vi "ScriptManager.vi"() -> ()   [LabVIEW 2021]
uses:
  <vilib>/Utility/miscctls.llb/LVSelectionTypeDef.ctl
  <vilib>/event_ctls.llb/eventvkey.ctl
  <vilib>/Utility/miscctls.llb/LVRectTypeDef.ctl
  <vilib>/Platform/browser.llb/Open URL in Default Browser (string).vi
  <vilib>/regexp/Match Regular Expression.xnode
  ScriptManager/ScriptManager.lvlib
  lib/UI/TreeControl/TreeControlLib.lvlib
panel:
  out "Dirty":refnum<vi>
  out "InifilePath":path
  out "PreviousSaveMode":string
  out "Allowed Parent Child":set{cluster{"Parent":i32, "Child":i32}}(c389)
  out "VKey":T1
  out "Edit Mode":enum16{"unknown", "inserting", "deleting"}(ring)
  out "Text.Selection":T2
  out "RedoBuffer":string[](array[string])
  out "UndoBuffer":string[](array[string])
  out "ItemTagToName":map{string, string}(c390)
  out "editor refs":refnum<vi>[](array[refnum])
  in  "Show Editor":bool
  in  "Tree":string(tree) caption="Tree (use right click menu to edit)"
  out "Last Modified":refnum<vi>
  in  "Exec":bool
  out "Modified":string
  in  "Description":string
  in  "Title":string
  in  "VI Property Picker":bool
  in  "Script":string
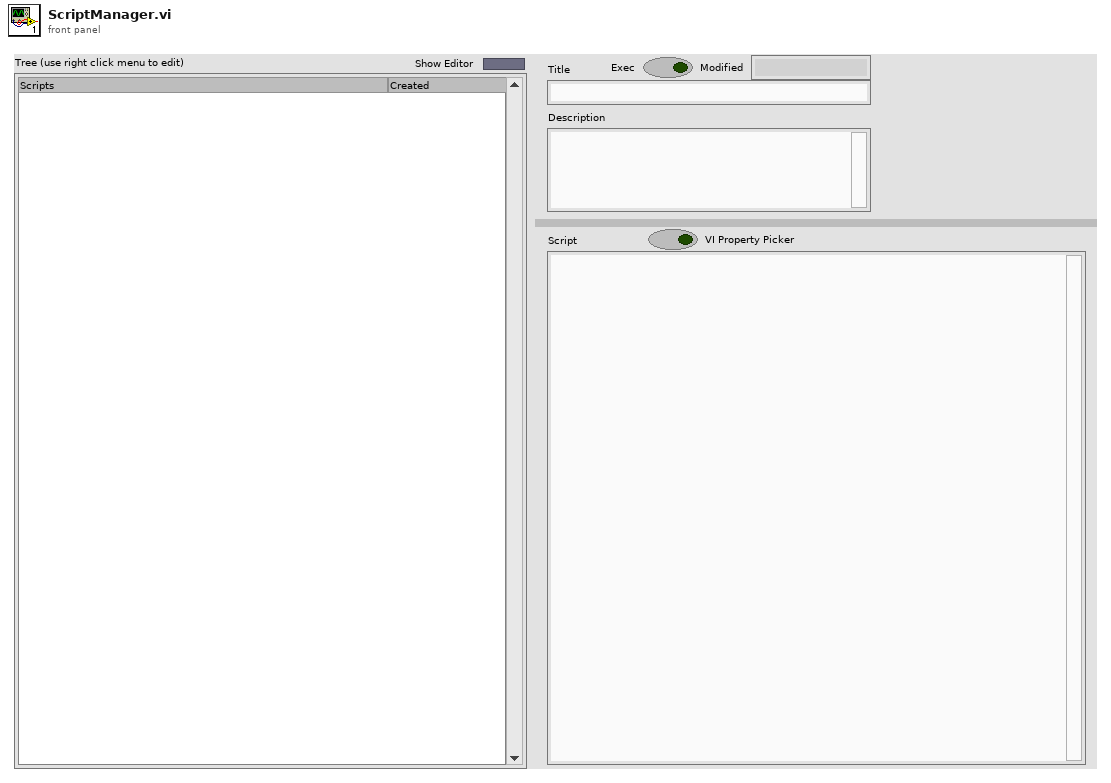
[diagram p1: front panel]
types:
  T1 = typedef "eventvkey.ctl" = enum16{"ASCII", "Enter", "Return", "Shift", "Ctrl", "Alt", "Cmd", "Opt", "Caps", "NumLock", "Clear", "Break", "Up", "Down", "Left", "Right", "Insert", "Delete", "Home", "End", "PageUp", "PageDown", "Escape", "Help", "Pause", "ScrollLock", "F1", "F2", "F3", "F4", "F5", "F6", "F7", "F8", "F9", "F10", "F11", "F12", "F13", "F14", "F15", "F16", "F17", "F18", "F19", "F20", "F21", "F22", "F23", "F24", "Play", "VolumeUp", "VolumeDown", "Mute", "Two Byte Char"}
  T2 = typedef "LVSelectionTypeDef.ctl" = cluster{"Selection Start":u32, "Selection End":u32}
  T3 = cluster{"Name":string, "Include Shift Key?":bool, "Include Ctrl Key?":bool, "Shortcut Key":string}[]
  T4 = enum32{"Invalid", "Standard", "Closed", "Hidden", "Minimized", "Maximized"}
  T5 = enum16{"open", "replace", "create", "open or create", "replace or create", "replace or create with confirmation"}
  T6 = typedef "LVRectTypeDef.ctl" = cluster{"Left":i16, "Top":i16, "Right":i16, "Bottom":i16}
  T7 = enum8{"Enabled", "Disabled", "Disabled and Grayed Out"}
  T8 = cluster{"[0]":i32, "[1]":i32, "[2]":i32, "[3]":i32, "[4]":i32}
  T9 = enum16{"Sticks Top/Left", "Sticks Bottom/Right", "Proportional"}
  T10 = typedef "LVPoint32TypeDef.ctl" = cluster{"Horizontal":i32, "Vertical":i32}
  T11 = typedef "LVRowAndColumnTypeDef.ctl" = cluster{"Row":i32, "Column":i32}
  T12 = typedef "lveventtype.ctl" = enum32{"Null", "Timeout", "Annotation Menu Selection", "Annotation Menu Selection?", "App Instance Close", "App Instance Close?", "Autoscale Range Change", "Bookmark Info Change", "Cell Edit", "Cell Edit?", "Cursor Grab", "Cursor Grab?", "Cursor Menu Selection", "Cursor Menu Selection?", "Cursor Move", "Cursor Release", "Data Change", "Direction Change", "Display State Change", "Drag Ended", "Drag Enter", "Drag Leave", "Drag Over", "Drag Source Update", "Drag Starting", "Drag Starting?", "Drop", "Exec State Change", "Key Down", "Key Down?", "Key Repeat", "Key Repeat?", "Key Up", "Listbox Double Click", "Menu Activation?", "Menu Selection (App)", "Menu Selection? (App)", "Menu Selection (User)", "Mouse Down", "Mouse Down?", "Mouse Enter", "Mouse Leave", "Mouse Move", "Mouse Up", "Mouse Wheel", "NI Security User Change (App)", "Pane Size", "Panel Close", "Panel Close?", "Panel Resize", "Plot Attribute Change", "Scale Range Change", "Shortcut Menu Activation?", "Shortcut Menu Selection (App)", "Shortcut Menu Selection? (App)", "Shortcut Menu Selection (User)", "Tree Double Click", "Tree Drag", "Tree Drag?", "Tree Drop", "Tree Drop?", "Tree Item Close", "Tree Item Close?", "Tree Item Open", "Tree Item Open?", "User Event", "Value Change"}
  T13 = cluster{"Shift":bool, "Ctrl":bool, "Alt":bool, "Cmd":bool, "Opt":bool}
  T14 = cluster{"Tag":string, "Symbol Index":i32, "Indent Level":i32, "Disabled?":bool, "In Symbol?":bool, "Position":enum16{"Top", "Center", "Bottom"}}
  T15 = enum32{"Bad", "Idle", "Run top level", "Running"}
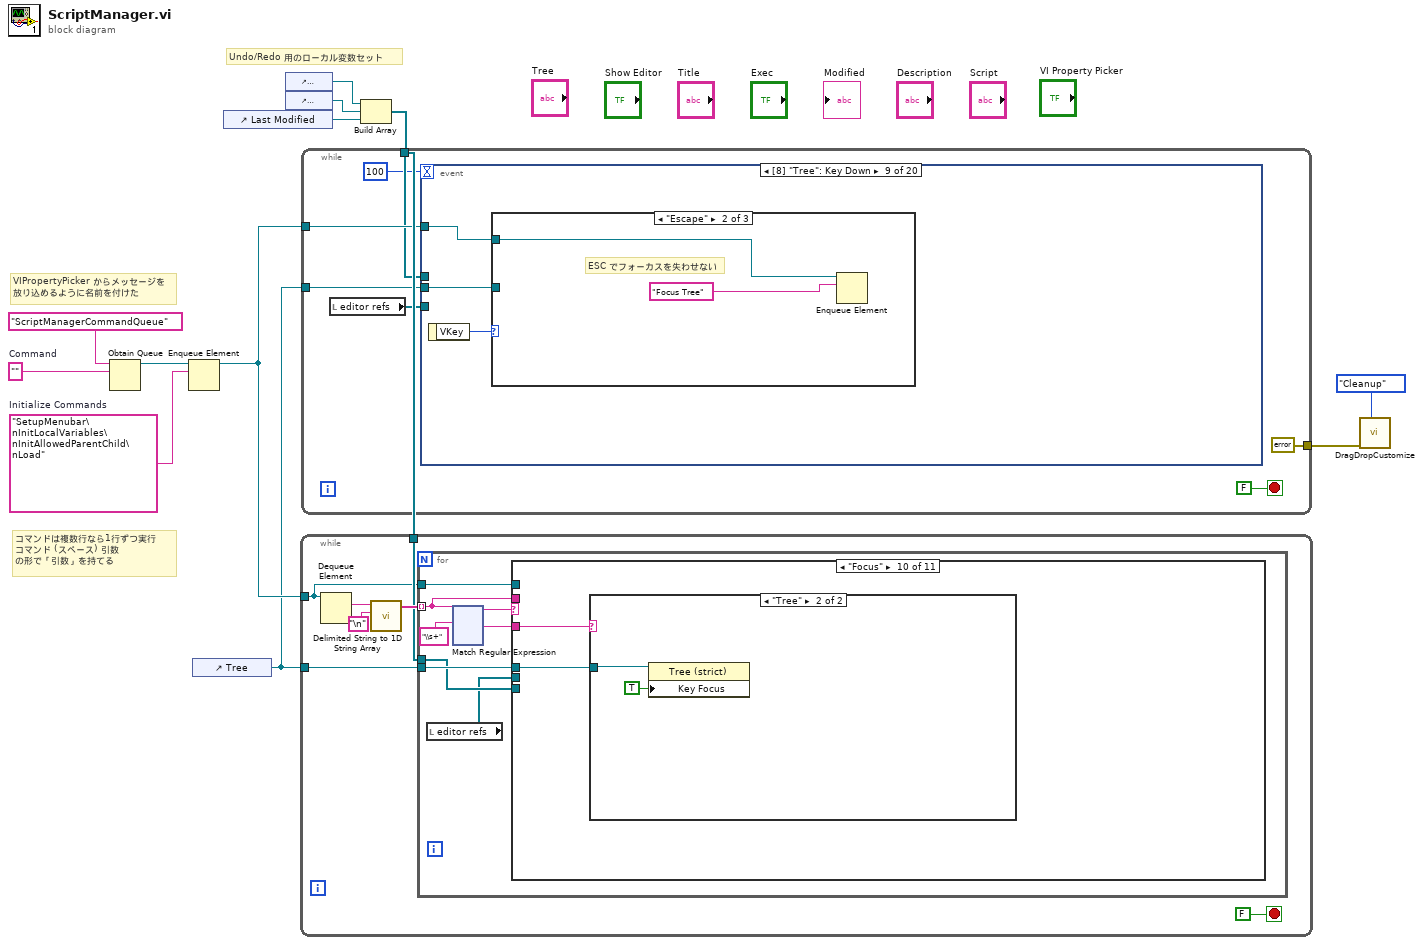
[diagram p0: block diagram]
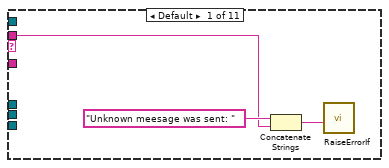
[diagram p2: hidden frame]
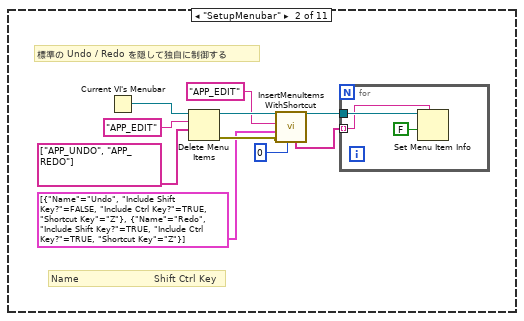
[diagram p3: hidden frame]
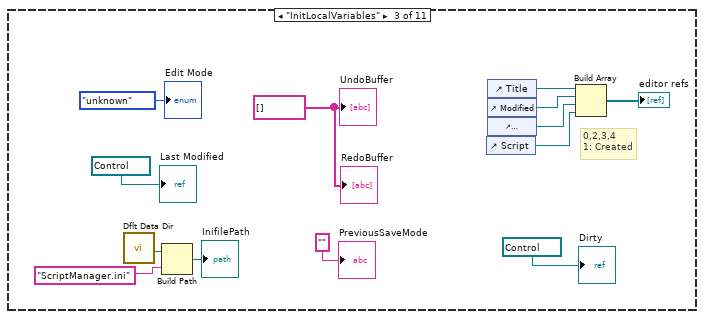
[diagram p4: hidden frame]
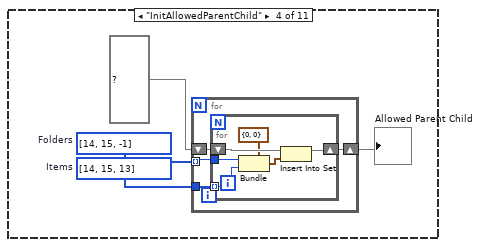
[diagram p5: hidden frame]
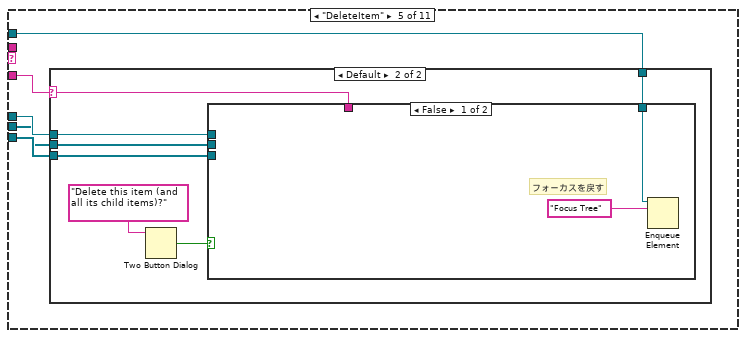
[diagram p6: hidden frame]
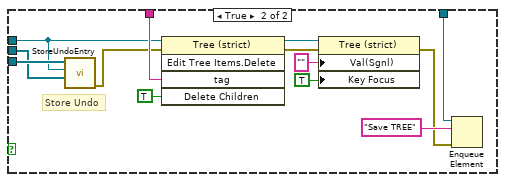
[diagram p8: hidden frame]
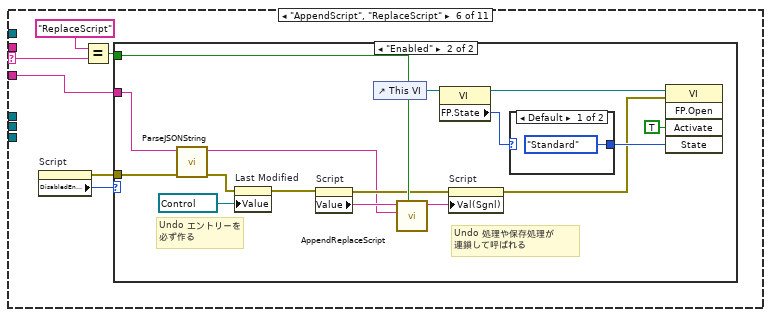
[diagram p9: hidden frame]
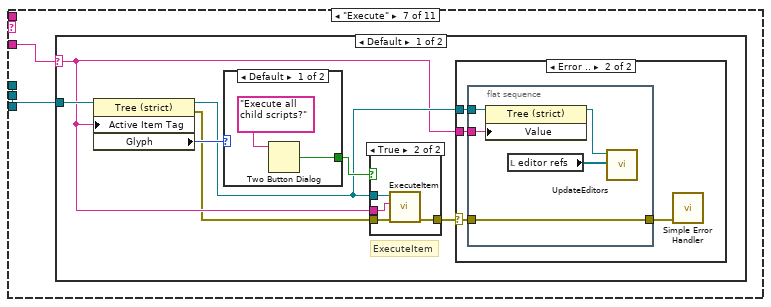
[diagram p12: hidden frame]
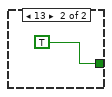
[diagram p15: hidden frame]
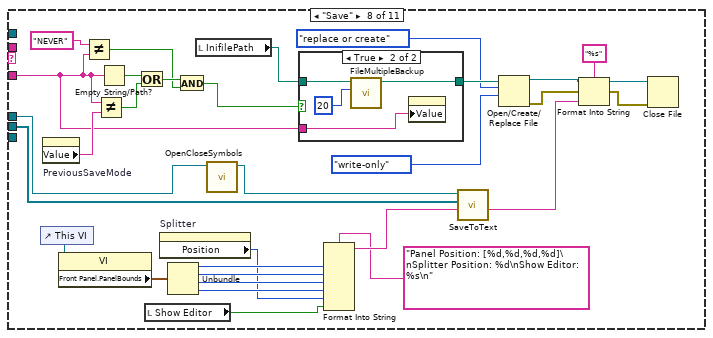
[diagram p17: hidden frame]
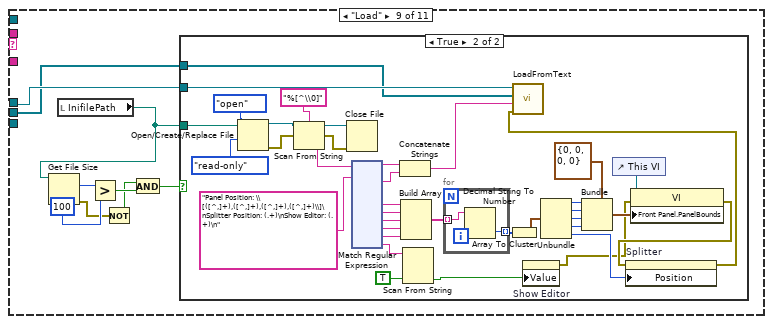
[diagram p19: hidden frame]
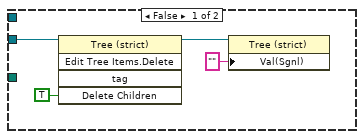
[diagram p20: hidden frame]
diagram:
  w7 = "SetupMenubar\nInitLocalVariables\nInitAllowedParentChild\nLoad"  # Initialize Commands
  w10 = ""  # Command
  # "Undo/Redo 用のローカル変数セット"
  # "コマンドは複数行なら1行ずつ実行\nコマンド (スペース) 引数\nの形で「引数」を持てる"
  # "VIPropertyPicker からメッセージを\n放り込めるように名前を付けた"
  n1 = Obtain Queue(name (unnamed)="ScriptManagerCommandQueue", element data type=w10) -> (queue out=w9:refnum<queue>)  [unwired: 3 in, 2 out]
  n2 = Enqueue Element(queue=w9, element=w7) -> (queue out=w8:refnum<queue>)  [unwired: 2 in, 2 out]
  n3 = control-ref of="Tree"() -> (w1:refnum<vi>)
  n4 = control-ref of="Last Modified"() -> (w2:refnum<vi>)
  n5 = control-ref of="UndoBuffer"() -> (w4:refnum<vi>)
  n6 = control-ref of="RedoBuffer"() -> (w5:refnum<vi>)
  n7 = Build Array(w4, w5, w2) -> (w3:refnum<vi>[])
  n8 = while {
    tunnel: w8 -> [w13]
    tunnel: w1 -> [w16]
    tunnel: w3 -> [w14]
    stop <- FALSE stop-if-true
    n9 = Dequeue Element(queue=w13) -> (element=w18:string)  [unwired: 2 in, 3 out]
    n10 = call <vilib>:"Delimited String to 1D String Array.vi"("delimiter"="\n", "delimited string"=w18) -> ("string array"=w17:string[])  [unwired: 9 in]
    n11 = for {
      tunnel: w17 -> [w20] mode=indexing
      tunnel: w16 -> [w24]
      tunnel: w14 -> [w23]
      tunnel: w13 -> [w22]
      n12 = local read "editor refs"() -> (w21:refnum<vi>[])
      n13 = xnode "Match Regular Expression"("input string"=w20, "regular expression"="\\s+") -> ("before match"=w26:string, "after match"=w25:string)  [unwired: 4 in, 3 out]
      n14 = case shown="\"Focus\"" w26 {
        selector: w26 -> [_ _ _ _ _ w217 _ _ _ _ _]
        tunnel: w25 -> [_ _ _ _ w192 w219 w240 w265 _ w478 _]
        tunnel: w24 -> [_ _ _ _ w191 _ w239 w269 w306 w477 _]
        tunnel: w20 -> [w146 _ _ _ _ _ _ _ _ _ _]
        tunnel: w23 -> [_ _ _ _ w190 _ _ _ _ _ _]
        tunnel: w21 -> [_ _ _ _ w189 _ _ w288 w305 _ _]
        tunnel: w22 -> [_ _ _ _ w188 _ _ _ _ _ _]
        frame Default {
          n15 = Concatenate Strings("Unknown meesage was sent: ", w146) -> (w145:string)
          n16 = call "RaiseErrorIf.vi"("error message"=w145) -> ()  [unwired: 10 in, 1 out]
        }
        frame "SetupMenubar" {
          # "標準の Undo / Redo を隠して独自に制御する"
          # "Name                         Shift Ctrl Key"
          n17 = Current VI's Menubar() -> (w153:refnum<k9>)
          n18 = Delete Menu Items(7:string[] ["APP_UNDO", "APP_REDO"], 8:"APP_EDIT", 9:w153) -> (0:w154:errorcluster, 3:w155:refnum<k9>)  [unwired: 1 in]
          n19 = call "InsertMenuItemsWithShortcut.vi"("Insert After (last)"=0, "error in (no error)"=w154, "Sub Items"=T3 [{"Name"="Undo", "Include Shift Key?"=FALSE, "Include Ctrl Key?"=TRUE, "Shortcut Key"="Z"}, {"Name"="Redo", "Include Shift Key?"=TRUE, "Include Ctrl Key?"=TRUE, "Shortcut Key"="Z"}] ("Menu Short Cut"), "Target Tag"="APP_EDIT", "menu ref"=w155) -> ("menu ref out"=w156:refnum<k9>, "Sub Item Names"=w157:string[])  [unwired: 3 in, 2 out]
          n20 = for {
            tunnel: w156 -> [w160]
            tunnel: w157 -> [w159] mode=indexing
            n21 = Set Menu Item Info(7:w159, 9:FALSE ("enabled"), 11:w160) -> ()  [unwired: 4 in, 2 out]
          }
        }
        frame "InitLocalVariables" {
          w166 = string[] [] ("UndoBuffer")
          # "0,2,3,4\n1: Created"
          n22 = call <vilib>:"Dflt Data Dir.vi"() -> ("App:Default Data Directory"=w164:path)
          n23 = Build Path(base path=w164, name or relative path="ScriptManager.ini") -> (appended path=→"InifilePath":path)
          n24 = control-ref of="Script"() -> (w169:refnum<vi>)
          n25 = control-ref of="Title"() -> (w168:refnum<vi>)
          n26 = control-ref of="Modified"() -> (w167:refnum<vi>)
          n27 = control-ref of="Description"() -> (w170:refnum<vi>)
          n28 = Build Array(w168, w167, w170, w169) -> (→"editor refs":refnum<vi>[])
          "Edit Mode" <- enum16{"unknown", "inserting", "deleting"}."unknown"
          "Last Modified" <- refnum<vi> refnum ("Last Modified")
          "UndoBuffer" <- w166
          "RedoBuffer" <- w166
          "PreviousSaveMode" <- "" ("PreviousSaveMode")
          "Dirty" <- refnum<vi> refnum ("Dirty")
        }
        frame "InitAllowedParentChild" {
          w177 = i32[] [14, 15, -1]  # Folders
          w176 = i32[] [14, 15, 13]  # Items
          n29 = for {
            tunnel: w177 -> [w179] mode=indexing
            tunnel: w176 -> [w181]
            shift-right: [w178] -> w174
            shift-left: set{cluster{"Parent":i32, "Child":i32}} {} ("Allowed Parent Child") -> [w180]
            n30 = for {
              tunnel: w181 -> [w187] mode=indexing
              tunnel: w179 -> [w186]
              shift-right: [w182] -> w178
              shift-left: w180 -> [w184]
              n31 = Bundle(cluster=cluster{"Parent":i32, "Child":i32} {"Parent"=0, "Child"=0} ("element"), "Parent"=w186, "Child"=w187) -> (w185:cluster{"Parent":i32, "Child":i32})
              n32 = Insert Into Set(10:w185, 11:w184) -> (3:w182:set{cluster{"Parent":i32, "Child":i32}})  [unwired: 1 out]
            }
          }
          "Allowed Parent Child" <- w174
        }
        frame "DeleteItem" {
          n33 = case shown="Default" w192 {
            selector: w192 -> [_ w198]
            tunnel: w191 -> [_ w199]
            tunnel: w190 -> [_ w195]
            tunnel: w189 -> [_ w194]
            tunnel: w188 -> [_ w193]
            frame "" {
            }
            frame Default {
              n34 = Two Button Dialog(message="Delete this item (and all its child items)?") -> (T button?=w196:bool)  [unwired: 2 in]
              n35 = case shown="False" w196 {
                tunnel: w199 -> [_ w207]
                tunnel: w198 -> [_ w213]
                tunnel: w195 -> [_ w208]
                tunnel: w194 -> [_ w206]
                tunnel: w193 -> [w200 w202]
                frame False {
                  # "フォーカスを戻す"
                  n36 = Enqueue Element(queue=w200, element="Focus Tree") -> ()  [unwired: 2 in, 3 out]
                }
                frame True {
                  # "Store Undo"
                  n37 = call "StoreUndoEntry.vi"("editor refs"=w206, "Tree"=w207, "UndoBuffer"=w208) -> ("error out"=w209:errorcluster)  [unwired: 8 in]
                  n38 = invoke class="Tree (strict)" method="Edit Tree Items.Delete"(reference=w207, error in=w209, "tag"=w213, "Delete Children"=TRUE ("Delete Children?")) -> (reference out=w212:refnum<vi>, error out=w211:errorcluster)  [unwired: 1 in, 3 out]
                  n39 = property class="Tree (strict)"(reference=w212, error in=w211, "Val(Sgnl)"="" ("Value"), "Key Focus"=TRUE) -> (error out=w203:errorcluster)  [unwired: 1 out]
                  n40 = Enqueue Element(queue=w202, element="Save TREE", error in (no error)=w203) -> ()  [unwired: 1 in, 3 out]
                }
              }
            }
          }
        }
        frame "AppendScript", "ReplaceScript" {
          n41 = property on="Script" class="Str"() -> (error out=w218:errorcluster, "DisabledEnum"=w220:T7)  [unwired: 2 in, 1 out]
          n42 = Equal?(x="ReplaceScript", y=w217) -> (x = y?=w215:bool)
          n43 = case shown="\"Enabled\"" w220 {
            tunnel: w219 -> [_ w236]
            tunnel: w218 -> [_ w234]
            tunnel: w215 -> [_ w227]
            frame Default {
            }
            frame "Enabled" {
              # "Undo エントリーを\n必ず作る"
              # "Undo 処理や保存処理が\n連鎖して呼ばれる"
              n44 = call "ParseJSONString.vi"("error in (no error)"=w234, "JSON string"=w236) -> ("error out"=w225:errorcluster, "string"=w221:string)  [unwired: 8 in]
              n45 = property on="Last Modified" class="LVObjRef (strict)"(error in=w225, "Value"=refnum<vi> refnum ("Last Modified")) -> (error out=w222:errorcluster)  [unwired: 1 in, 1 out]
              n46 = property on="Script" class="Str"(error in=w222) -> (error out=w226:errorcluster, "Value"=w228:string)  [unwired: 1 in, 1 out]
              n47 = control-ref of="This VI"() -> (w233:refnum<vi>)
              n48 = call "AppendReplaceScript.vi"("Replace"=w227, "New Script"=w221, "Old Script"=w228) -> ("Result"=w235:string)  [unwired: 8 in]
              n49 = property class="VI"(reference=w233) -> (reference out=w231:refnum<vi>, "FP.State"=w230:T4)  [unwired: 1 in, 1 out]
              n50 = property on="Script" class="Str"(error in=w226, "Val(Sgnl)"=w235) -> (error out=w223:errorcluster)  [unwired: 1 in, 1 out]
              n51 = case shown="Default" w230 {
                selector: w230 -> [_ w238]
                tunnel: [T4."Standard" ("State") w238] -> w229
                frame Default {
                }
                frame "Standard", "Maximized" {
                }
              }
              n52 = invoke class="VI" method="FP.Open"(reference=w231, error in=w223, "Activate"=TRUE ("Activate?"), "State"=w229) -> ()  [unwired: 1 in, 5 out]
            }
          }
        }
        frame "Execute" {
          n53 = case shown="Default" w240 {
            selector: w240 -> [w242 _]
            tunnel: w239 -> [w247 _]
            frame Default {
              # "ExecuteItem"
              n54 = property class="Tree (strict)"(reference=w247, "Active Item Tag"=w242) -> (reference out=w243:refnum<vi>, error out=w241:errorcluster, "Glyph"=w246:i32)  [unwired: 1 in]
              n55 = case shown="Default" w246 {
                tunnel: [w262 TRUE ("T button?")] -> w245
                frame Default {
                  n56 = Two Button Dialog(message="Execute all child scripts?") -> (T button?=w262:bool)  [unwired: 2 in]
                }
                frame 13 {
                }
              }
              n57 = case shown="True" w245 {
                tunnel: w243 -> [_ w261]
                tunnel: w242 -> [_ w260]
                tunnel: [w257 w259] -> w244
                tunnel: w241 -> [w257 w258]
                frame False {
                }
                frame True {
                  n58 = call "ExecuteItem.vi"("error in (no error)"=w258, "Tag"=w260, "TreeControl in"=w261) -> ("error out"=w259:errorcluster)  [unwired: 8 in]
                }
              }
              n59 = case shown="Error .." w244 {
                selector: w244 -> [_ w249]
                tunnel: w243 -> [_ w251]
                tunnel: w242 -> [_ w250]
                frame No Error {
                }
                frame Error {
                  n60 = flat-sequence {
                    tunnel: w251 -> [w256]
                    tunnel: w250 -> [w255]
                    tunnel: w249 -> [w252]
                    tunnel: [w252] -> w248
                    frame #0 {
                      n61 = property class="Tree (strict)"(reference=w256, "Value"=w255) -> (reference out=w254:refnum<vi>)  [unwired: 1 in, 1 out]
                      n62 = local read "editor refs"() -> (w253:refnum<vi>[])
                      n63 = call "UpdateEditors.vi"("Array"=w253, "TreeControl in"=w254) -> ()  [unwired: 9 in, 1 out]
                    }
                  }
                  n64 = call <vilib>:"Simple Error Handler.vi"("error in (no error)"=w248) -> ()  [unwired: 4 in, 5 out]
                }
              }
            }
            frame "" {
            }
          }
        }
        frame "Save" {
          n65 = control-ref of="This VI"() -> (w283:refnum<vi>)
          n66 = property on="PreviousSaveMode" class="Str"() -> ("Value"=w267:string)  [unwired: 2 in, 2 out]
          n67 = property class="VI"(reference=w283) -> ("Front Panel.PanelBounds"=w282:T6)  [unwired: 1 in, 2 out]
          n68 = Not Equal?(x="NEVER", y=w265) -> (x != y?=w270:bool)
          n69 = Not Equal?(x=w265, y=w267) -> (x != y?=w294:bool)
          n70 = Empty String/Path?(string/path=w265) -> (empty?=w295:bool)
          n71 = Or(x=w295, y=w294) -> (x .or. y?=w292:bool)
          n72 = local read "Show Editor"() -> (w276:bool)
          n73 = property on="Splitter" class="Splitter"() -> ("Position"=w277:i32)  [unwired: 2 in, 2 out]
          n74 = Unbundle(w282) -> ("Left"=w281:i16, "Top"=w280:i16, "Right"=w279:i16, "Bottom"=w278:i16)
          n75 = And(x=w292, y=w270) -> (x .and. y?=w271:bool)
          n76 = local read "InifilePath"() -> (w293:path)
          n77 = call "OpenCloseSymbols.vi"("Tree ref"=w269) -> ("Tree ref out"=w268:refnum<vi>)  [unwired: 9 in, 1 out]
          n78 = case shown="True" w271 {
            tunnel: w293 -> [w296 w299]
            tunnel: [w296 w298] -> w291
            tunnel: w265 -> [_ w297]
            frame False {
            }
            frame True {
              n79 = call "FileMultipleBackup.vi"("Number of Backups"=20, "File path"=w299) -> ("File path out"=w298:path)  [unwired: 9 in]
              n80 = property on="PreviousSaveMode" class="Str"("Value"=w297) -> ()  [unwired: 2 in, 2 out]
            }
          }
          n81 = Format Into String(format string="Panel Position: [%d,%d,%d,%d]\nSplitter Position: %d\nShow Editor: %s\n", w281, w280, w279, w278, w277, w276) -> (resulting string=w275:string)  [unwired: 2 in, 1 out]
          n82 = call "SaveToText.vi"("Additional Header"=w275, "editor refs"=w288, "Tree ref"=w268) -> ("String"=w285:string)  [unwired: 7 in, 1 out]
          n83 = Open/Create/Replace File(file path (use dialog)=w291, operation (0:open)=T5."replace or create", access (0:read/write)=enum16{"read/write", "read-only", "write-only"}."write-only") -> (refnum out=w287:refnum<file>, error out=w286:errorcluster)  [unwired: 3 in, 1 out]
          n84 = Format Into String(format string="%s", initial string=w287, error in=w286, w285) -> (resulting string=w273:refnum<file>, error out=w274:errorcluster)
          n85 = Close File(refnum=w273, error in=w274) -> ()  [unwired: 2 out]
        }
        frame "Load" {
          n86 = local read "InifilePath"() -> (w301:path)
          n87 = Get File Size(file=w301) -> (size (in bytes)=w309:i64, 0:w303:errorcluster)  [unwired: 1 in, 1 out]
          n88 = Greater?(x=w309, y=i64 100) -> (0:w307:bool)
          n89 = Not(x=w303) -> (.not. x?=w302:bool)
          n90 = And(x=w302, y=w307) -> (x .and. y?=w304:bool)
          n91 = case shown="True" w304 {
            tunnel: w301 -> [_ w344]
            tunnel: w306 -> [w313 w317]
            tunnel: w305 -> [_ w316]
            frame False {
              n92 = invoke class="Tree (strict)" method="Edit Tree Items.Delete"(reference=w313, "Delete Children"=TRUE ("Delete Children?")) -> (reference out=w312:refnum<vi>)  [unwired: 3 in, 4 out]
              n93 = property class="Tree (strict)"(reference=w312, "Val(Sgnl)"="" ("Value (Signaling)")) -> ()  [unwired: 1 in, 2 out]
            }
            frame True {
              n94 = Open/Create/Replace File(file path (use dialog)=w344, operation (0:open)=T5."open", access (0:read/write)=enum16{"read/write", "read-only", "write-only"}."read-only") -> (refnum out=w347:refnum<file>, error out=w348:errorcluster)  [unwired: 3 in, 1 out]
              n95 = Scan From String("%[^\\0]" ("format string"), w347, w348) -> (w350:refnum<file>, w349:errorcluster, output 1=w341:string)  [unwired: 1 in]
              n96 = Close File(refnum=w350, error in=w349) -> ()  [unwired: 2 out]
              n97 = xnode "Match Regular Expression"("input string"=w341, "regular expression"="Panel Position: \\[([^,]+),([^,]+),([^,]+),([^,]+)\\]\nSplitter Position: (.+)\nShow Editor: (.+)\n" ("format string")) -> ("before match"=w334:string, "after match"=w333:string, "submatch 1"=w340:string, "submatch 2"=w339:string, "submatch 3"=w338:string, "submatch 4"=w337:string, "submatch 5"=w336:string, "submatch 6"=w323:string)  [unwired: 4 in, 3 out]
              n98 = Concatenate Strings(w334, w333) -> (w318:string)
              n99 = Build Array(w340, w339, w338, w337, w336) -> (w335:string[])
              n100 = Scan From String(input string=w323, default 1=TRUE) -> (output 1=w321:bool)  [unwired: 3 in, 3 out]
              n101 = for {
                tunnel: w335 -> [w352] mode=indexing
                tunnel: [w351] -> w332 mode=indexing
                n102 = Decimal String To Number(string=w352) -> (number=w351:i32)  [unwired: 2 in, 1 out]
              }
              n103 = Array To Cluster(array=w332) -> (cluster=w331:T8)
              n104 = property on="Show Editor" class="Bool (strict)"("Value"=w321) -> (error out=w315:errorcluster)  [unwired: 2 in, 1 out]
              n105 = Unbundle(w331) -> ("[0]"=w329:i32, "[1]"=w328:i32, "[2]"=w327:i32, "[3]"=w326:i32, "[4]"=w320:i32)
              n106 = Bundle(cluster=T6 {"Left"=0, "Top"=0, "Right"=0, "Bottom"=0} ("Front Panel Window:Panel Bounds"), "Left"=w329, "Top"=w328, "Right"=w327, "Bottom"=w326) -> (w325:T6)
              n107 = control-ref of="This VI"() -> (w324:refnum<vi>)
              n108 = property class="VI"(reference=w324, error in=w315, "Front Panel.PanelBounds"=w325) -> (error out=w319:errorcluster)  [unwired: 1 out]
              n109 = property on="Splitter" class="Splitter"(error in=w319, "Position"=w320) -> (error out=w314:errorcluster)  [unwired: 1 in, 1 out]
              n110 = call "LoadFromText.vi"("error in"=w314, "String"=w318, "editor refs"=w316, "Tree ref"=w317) -> ()  [unwired: 6 in, 2 out]
            }
          }
        }
        frame "Focus" {
          n111 = case shown="\"Tree\"" w478 {
            tunnel: w477 -> [_ w480]
            frame Default {
            }
            frame "Tree" {
              n112 = property class="Tree (strict)"(reference=w480, "Key Focus"=TRUE) -> ()  [unwired: 1 in, 2 out]
            }
          }
        }
        frame "" {
        }
      }
    }
  }
  n113 = while {
    tunnel: [errorcluster {"status"=FALSE, "code"=0, "source"=""} ("error in (no error)")] -> w11
    tunnel: w8 -> [w485]
    tunnel: w3 -> [w483]
    tunnel: w1 -> [w482]
    stop <- FALSE stop-if-true
    n114 = local read "editor refs"() -> (w484:refnum<vi>[])
    n115 = event shown="[8] \"Tree\": Key Down" {
      selector: _ -> [_ _ _ _ _ _ _ _ _ _ _ _ _ _ _ _ _ _ _ _]
      dyn-events: _ -> [_ _ _ _ _ _ _ _ _ _ _ _ _ _ _ _ _ _ _ _]
      timeout: 100 -> [_ _ _ _ _ _ _ _ _ _ _ _ _ _ _ _ _ _ _ _]
      tunnel: w482 -> [w492 _ _ _ w564 w583 _ w638 w657 w683 _ _ _ w732 _ _ _ _ _ _]
      tunnel: w485 -> [w490 w527 w540 w542 _ w582 _ w636 w658 w679 _ w709 _ w729 _ _ _ w770 w778 _]
      tunnel: w484 -> [w491 _ _ _ _ w578 _ w637 _ w682 _ _ _ w727 _ _ _ _ _ _]
      tunnel: w483 -> [w493 _ _ _ _ w577 _ w639 _ w684 _ _ _ w728 _ _ _ _ _ _]
      event Timeout {
        n116 = event-data() -> ()  [unwired: 1 in, 1 out]
        n117 = local read "Dirty"() -> (w488:refnum<vi>)
        n118 = Not A Number/Path/Refnum?(number/path/refnum=w488) -> (NaN/Path/Refnum?=w489:bool)
        n119 = case shown="False" w489 {
          tunnel: w493 -> [w501 _]
          tunnel: w492 -> [w500 _]
          tunnel: w491 -> [w499 _]
          tunnel: w490 -> [w496 _]
          tunnel: w488 -> [w495 _]
          frame False {
            n120 = local read "Text.Selection"() -> (w497:T2)
            n121 = call "StoreUndoEntry.vi"("Text.Selection"=w497, "Changed Editor"=w495, "editor refs"=w499, "Tree"=w500, "UndoBuffer"=w501) -> ("error out"=w498:errorcluster)  [unwired: 6 in]
            n122 = property class="Tree (strict)"(reference=w500, error in=w498) -> (reference out=w503:refnum<vi>, error out=w502:errorcluster, "Value"=w504:string)
            n123 = local write "Dirty"(refnum<vi> refnum ("Dirty")) -> ()
            n124 = case shown="Default" w504 {
              selector: w504 -> [_ w510]
              tunnel: w503 -> [_ w509]
              tunnel: w502 -> [_ w508]
              tunnel: w496 -> [_ w505]
              frame "" {
              }
              frame Default {
                n125 = Format Date/Time String(time format string (%c)="%Y-%m-%d %H:%M:%S") -> (date/time string=w511:string)  [unwired: 2 in]
                n126 = local read "Description"() -> (w515:string)
                n127 = local read "Script"() -> (w514:string)
                n128 = local read "Title"() -> (w516:string)
                n129 = local write "Modified"(w511) -> ()
                n130 = Build Array(w516, w511, w515, w514) -> (w513:string[])
                n131 = for {
                  shift-right: [w522] -> _
                  shift-left: w509 -> [w524]
                  shift-right: [w523] -> w506
                  shift-left: w508 -> [w521]
                  tunnel: i32[] [0, 2, 3, 4] -> [w520] mode=indexing
                  tunnel: w513 -> [w519] mode=indexing
                  tunnel: w510 -> [w518]
                  n132 = property class="Tree (strict)"(reference=w524, error in=w521, "Active Item Tag"=w518, "ActiveColNum"=w520, "Cell String"=w519) -> (reference out=w522:refnum<vi>, error out=w523:errorcluster)
                }
                n133 = Enqueue Element(queue=w505, element="Save EDIT", error in (no error)=w506) -> ()  [unwired: 1 in, 3 out]
              }
            }
          }
          frame True {
          }
        }
      }
      event Pane Size {
        # "ウィンドウサイズを保存する\n（バックアップは取らない）"
        # "Pane の幅が変わったら Col 0 の幅を変える"
        n134 = event-data() -> ("OldBnds.Right"=w537:i16, "OldBnds.Left"=w536:i16, "NewBnds.Right"=w535:i16, "NewBnds.Left"=w534:i16)  [unwired: 1 in]
        n135 = property on="Tree" class="Tree (strict)"("ActiveColNum"=0 ("Active Cell:Active Column Number")) -> ("Width"=w531:i32)  [unwired: 2 in, 2 out]
        n136 = Subtract(x=w537, y=w536) -> (x-y=w532:i16)
        n137 = Subtract(x=w535, y=w534) -> (x-y=w533:i16)
        n138 = Subtract(x=w533, y=w532) -> (x-y=w530:i16)
        n139 = Add(x=w531, y=w530) -> (x+y=w529:i32)
        n140 = property on="Tree" class="Tree (strict)"("ActiveColNum"=0 ("Active Cell:Active Column Number"), "Width"=w529) -> (error out=w526:errorcluster)  [unwired: 2 in, 1 out]
        n141 = Enqueue Element(queue=w527, element="Save NEVER", error in (no error)=w526) -> ()  [unwired: 1 in, 3 out]
      }
      event Panel Resize {
        # "ウィンドウサイズを保存する\n（バックアップは取らない）"
        n142 = event-data() -> ()  [unwired: 1 in, 2 out]
        n143 = Enqueue Element(queue=w540, element="Save NEVER") -> ()  [unwired: 2 in, 3 out]
      }
      event "Show Editor": Value Change {
        # "ウィンドウサイズの変更"
        # "ウィンドウサイズを保存する\n（バックアップは取らない）"
        n144 = event-data() -> ("NewVal"=w548:bool)  [unwired: 1 in]
        n145 = property on="Splitter" class="Splitter"("Sizing"=T9."Sticks Top/Left") -> (error out=w546:errorcluster)  [unwired: 2 in, 1 out]
        n146 = property on="Pane" class="Pane"(error in=w546) -> ("Width"=w551:u32)  [unwired: 1 in, 2 out]
        n147 = Select(t=u32 500, s=w548, f=u32 100 ("y")) -> (s? t:f=w554:u32)
        n148 = control-ref of="This VI"() -> (w556:refnum<vi>)
        n149 = Add(x=w551, y=w554) -> (x+y=w555:u32)
        n150 = Select(t=T9."Sticks Top/Left" ("Sizing"), s=w548, f=T9."Sticks Bottom/Right" ("Sizing")) -> (s? t:f=w545:T9)
        n151 = call "SetFrontPanelSize.vi"("Width (0: unchange)"=w555, "VI Reference"=w556) -> ("error out"=w544:errorcluster)  [unwired: 8 in, 1 out]
        n152 = flat-sequence {
          tunnel: w545 -> [w558]
          tunnel: w544 -> [_]
          tunnel: [w557] -> w541
          frame #0 {
            n153 = property on="Splitter" class="Splitter"("Sizing"=w558) -> (error out=w557:errorcluster)  [unwired: 2 in, 1 out]
          }
        }
        n154 = Enqueue Element(queue=w542, element="Save NEVER", error in (no error)=w541) -> ()  [unwired: 1 in, 3 out]
      }
      event "Tree": Shortcut Menu Activation? {
        # "クリックされた項目があればそれを選択\nクリックされた項目がなければ選択済み項目を使う"
        # "クリックされた項目を得る"
        # "メニューを設定"
        n155 = event-data() -> ("MenuRef"=w566:refnum<k9>, "Coords"=w565:T10)  [unwired: 1 in]
        n156 = invoke class="Tree (strict)" method="Point To Row Column"(reference=w564, "Point"=w565) -> (reference out=w562:refnum<vi>, error out=w560:errorcluster, "Tag"=w563:string)  [unwired: 6 in, 5 out]
        n157 = case shown="Default" w563 {
          selector: w563 -> [w567 _]
          tunnel: w562 -> [w568 w576]
          tunnel: [w567 w571] -> w561
          tunnel: w560 -> [_ w569]
          frame Default {
            n158 = property class="Tree (strict)"(reference=w568, "Value"=w567, "FocusItem"=w567) -> ()  [unwired: 1 in, 2 out]
          }
          frame "" {
            # "存在しない\nなら空文字"
            n159 = property class="Tree (strict)"(reference=w576, error in=w569) -> (reference out=w575:refnum<vi>, error out=w574:errorcluster, "Value"=w572:string)
            n160 = property class="Tree (strict)"(reference=w575, error in=w574, "Active Item Tag"=w572) -> (error out=w573:errorcluster)  [unwired: 1 out]
            n161 = Select(t="", s=w573, f=w572) -> (s? t:f=w571:string)
          }
        }
        n162 = call "TreePopup.vi"("TreeView Value"=w561, "Menu in"=w566) -> ("ItemTagToName"=→"ItemTagToName":map{string, string})  [unwired: 9 in]
        n163 = event-data() -> ()  [unwired: 2 in, 1 out]
      }
      event "Tree": Shortcut Menu Selection (User) {
        n164 = event-data() -> ("ItemTag"=w579:string)  [unwired: 1 in]
        n165 = local read "ItemTagToName"() -> (w581:map{string, string})
        n166 = Look In Map(map=w581, key=w579) -> (value=w580:string)  [unwired: 1 in, 1 out]
        n167 = case shown="\"New Script\"" w580 {
          tunnel: w583 -> [_ w589 w597 w605 w621 _]
          tunnel: w582 -> [_ w592 w598 w608 w625 _]
          tunnel: w579 -> [w584 _ _ _ _ _]
          tunnel: w578 -> [_ w588 w595 w606 _ _]
          tunnel: w577 -> [_ w590 w596 w607 _ _]
          frame Default {
            n168 = Format Into String(format string="Unknown menu \"%s\" called.", w584) -> (resulting string=w585:string)  [unwired: 2 in, 1 out]
            n169 = call "RaiseErrorIf.vi"("error message"=w585) -> ()  [unwired: 10 in, 1 out]
          }
          frame "New Script" {
            n170 = call "StoreUndoEntry.vi"("editor refs"=w588, "Tree"=w589, "UndoBuffer"=w590) -> ("error out"=w587:errorcluster)  [unwired: 8 in]
            n171 = call "NewItem.vi"("error in (no error)"=w587, "TreeControl in"=w589) -> ("error out"=w593:errorcluster)  [unwired: 8 in, 1 out]
            n172 = Enqueue Element(queue=w592, element="Save TREE", error in (no error)=w593) -> ()  [unwired: 1 in, 3 out]
          }
          frame "New Folder" {
            n173 = call "StoreUndoEntry.vi"("editor refs"=w595, "Tree"=w597, "UndoBuffer"=w596) -> ("error out"=w594:errorcluster)  [unwired: 8 in]
            n174 = call "NewItem.vi"("error in (no error)"=w594, "Folder?"=TRUE, "TreeControl in"=w597) -> ("error out"=w599:errorcluster)  [unwired: 7 in, 1 out]
            n175 = Enqueue Element(queue=w598, element="Save TREE", error in (no error)=w599) -> ()  [unwired: 1 in, 3 out]
          }
          frame "Duplicate" {
            n176 = property class="Tree (strict)"(reference=w605) -> (reference out=w604:refnum<vi>, error out=w603:errorcluster, "Value"=w602:string)  [unwired: 1 in]
            n177 = case shown="Default" w602 {
              selector: w602 -> [_ w609]
              tunnel: w608 -> [_ w617]
              tunnel: w607 -> [_ w616]
              tunnel: w606 -> [_ w615]
              tunnel: w605 -> [_ w614]
              tunnel: w604 -> [_ w612]
              tunnel: w603 -> [_ w611]
              frame "" {
              }
              frame Default {
                n178 = call "StoreUndoEntry.vi"("error in (no error)"=w611, "editor refs"=w615, "Tree"=w614, "UndoBuffer"=w616) -> ("error out"=w610:errorcluster)  [unwired: 7 in]
                n179 = call "DuplicateItem.vi"("error in (no error)"=w610, "ItemTag"=w609, "TreeControl in"=w612) -> ("error out"=w613:errorcluster)  [unwired: 8 in]
                n180 = Enqueue Element(queue=w617, element="Save TREE", error in (no error)=w613) -> ()  [unwired: 1 in, 3 out]
              }
            }
          }
          frame "Delete" {
            n181 = property class="Tree (strict)"(reference=w621) -> (error out=w620:errorcluster, "Value"=w624:string)  [unwired: 1 in, 1 out]
            n182 = Format Into String(format string="DeleteItem %s", error in=w620, w624) -> (resulting string=w623:string, error out=w619:errorcluster)  [unwired: 1 in]
            n183 = Enqueue Element(queue=w625, element=w623, error in (no error)=w619) -> ()  [unwired: 1 in, 3 out]
          }
          frame "Help" {
            n184 = call-poly <vilib>:"Open URL in Default Browser.vi"("URL"="https://github.com/osamutake/labviewfolder/tree/main/utilities#scriptmanagervi") -> ()  [unwired: 5 in, 2 out]
          }
        }
      }
      event "UndoBuffer", "RedoBuffer": Value Change {
        # "Undo / Redo メニューの \nEnable /Disable を設定"
        n185 = event-data() -> ()  [unwired: 1 in, 6 out]
        n186 = local read "UndoBuffer"() -> (w635:string[])
        n187 = local read "RedoBuffer"() -> (w634:string[])
        n188 = Array Size(array=w635) -> (size(s)=w629:i32)
        n189 = Array Size(array=w634) -> (size(s)=w630:i32)
        n190 = Greater Than 0?(x=w629) -> (x > 0?=w628:bool)
        n191 = Greater Than 0?(x=w630) -> (x > 0?=w627:bool)
        n192 = Current VI's Menubar() -> (w631:refnum<k9>)
        n193 = Set Menu Item Info(7:"Undo" ("item tag"), 9:w628, 11:w631) -> ()  [unwired: 4 in, 2 out]
        n194 = Set Menu Item Info(7:"Redo" ("item tag"), 9:w627, 11:w631) -> ()  [unwired: 4 in, 2 out]
      }
      event Menu Selection (User) {
        n195 = event-data() -> ("ItemTag"=w640:string)  [unwired: 1 in]
        n196 = case shown="\"Undo\"" w640 {
          tunnel: w639 -> [_ w646 w652]
          tunnel: w638 -> [_ w648 w656]
          tunnel: w637 -> [_ w647 w655]
          tunnel: w636 -> [_ w642 w650]
          frame Default {
            n197 = call "RaiseErrorIf.vi"("error message"="Unknown menu item.") -> ()  [unwired: 10 in, 1 out]
          }
          frame "Undo" {
            n198 = call "UndoRedo.vi"("editor refs"=w647, "Tree"=w648, "UndoBuffer"=w646) -> ("error out"=w643:errorcluster)  [unwired: 8 in]
            n199 = local write "Last Modified"(refnum<vi> refnum ("Last Modified")) -> ()
            n200 = Enqueue Element(queue=w642, element="Save NEVER", error in (no error)=w643) -> ()  [unwired: 1 in, 3 out]
          }
          frame "Redo" {
            n201 = call "UndoRedo.vi"("Undo (T)"=FALSE, "editor refs"=w655, "Tree"=w656, "UndoBuffer"=w652) -> ("error out"=w649:errorcluster)  [unwired: 7 in]
            n202 = local write "Last Modified"(refnum<vi> refnum ("Last Modified")) -> ()
            n203 = Enqueue Element(queue=w650, element="Save NEVER", error in (no error)=w649) -> ()  [unwired: 1 in, 3 out]
          }
        }
      }
      event "Tree": Key Down {
        n204 = event-data() -> ("VKey"=w659:T1)  [unwired: 1 in]
        n205 = case shown="\"Escape\"" w659 {
          tunnel: w658 -> [w669 w676 _]
          tunnel: w657 -> [w668 _ _]
          frame "Delete" {
            w664 = -2 ("x")
            # "項目が編集中でないことを確認"
            n206 = property class="Tree (strict)"(reference=w668) -> ("Value"=w670:string, "EditPos"=w667:T11)  [unwired: 1 in, 2 out]
            n207 = Unbundle(w667) -> ("Row"=w666:i32, "Column"=w665:i32)
            n208 = Equal?(x=w664, y=w666) -> (x = y?=w663:bool)
            n209 = Equal?(x=w664, y=w665) -> (x = y?=w662:bool)
            n210 = Or(x=w663, y=w662) -> (x .or. y?=w661:bool)
            n211 = case shown="True" w661 {
              tunnel: w670 -> [_ w674]
              tunnel: w669 -> [_ w672]
              tunnel: "DeleteItem " ("string") -> [_ w671]
              frame False {
              }
              frame True {
                n212 = Concatenate Strings(w671, w674) -> (w673:string)
                n213 = Enqueue Element(queue=w672, element=w673) -> ()  [unwired: 2 in, 3 out]
              }
            }
          }
          frame "Escape" {
            # "ESC でフォーカスを失わせない"
            n214 = Enqueue Element(queue=w676, element="Focus Tree" ("string")) -> ()  [unwired: 2 in, 3 out]
          }
          frame Default {
          }
        }
      }
      event "Tree": event type 3.0.xa000003a; "Tree": Drop {
        n215 = event-data() -> ("Type"=w677:T12, "CtlRef"=w696:refnum<vi>, "Coords"=w695:T10, "PlatMods"=w689:T13, "Available Data Names"=w688:string[])  [unwired: 1 in]
        n216 = case shown="\"Drop\"" w677 {
          tunnel: w684 -> [_ w703]
          tunnel: w683 -> [_ w702]
          tunnel: w682 -> [_ w701]
          tunnel: [_ w700] -> w681
          frame "Null", Default {
          }
          frame "Drop" {
            # "Store Undo Entry"
            n217 = call "StoreUndoEntry.vi"("editor refs"=w701, "Tree"=w702, "UndoBuffer"=w703) -> ("error out"=w700:errorcluster)  [unwired: 8 in]
          }
        }
        n218 = local read "Allowed Parent Child"() -> (w680:set{cluster{"Parent":i32, "Child":i32}})
        n219 = call "DragDropCustomize.vi"("Set Cursor (T)"=FALSE, "Function"=enum16{"Event", "Cleanup"}."Event", "error in (no error)"=w681, "Coords"=w695, "CtlRef"=w696, "Event Type"=w677) -> ("error out"=w690:errorcluster, "InBounds"=w691:bool, "CtlRef out"=w692:refnum<vi>, "Drag Status"=w693:T14, "Bar Cursor ID"=w685:refnum<k1>)  [unwired: 1 in]
        n220 = call "DragDropMoveCopy.vi"("Type"=w677, "Allowed Parent Child"=w680, "Bar Cursor ID"=w685, "Drag Status"=w693, "CtlRef"=w692, "InBounds in"=w691, "error in"=w690, "PlatMods"=w689, "Available Data Names"=w688) -> ("Accepted?"=w687:bool, "error out"=w678:errorcluster)  [unwired: 1 in, 4 out]
        n221 = case shown="\"Drop\"" w677 {
          tunnel: w679 -> [_ w698]
          tunnel: w678 -> [_ w697]
          frame Default {
          }
          frame "Drop" {
            n222 = Enqueue Element(queue=w698, element="Save TREE", error in (no error)=w697) -> ()  [unwired: 1 in, 3 out]
          }
        }
        n223 = event-data("Accepted?"=w687) -> ()  [unwired: 1 in, 1 out]
      }
      event "Tree": Drag Ended {
        n224 = event-data() -> ("Type"=w705:T12, "CtlRef"=w704:refnum<vi>)  [unwired: 1 in, 3 out]
        n225 = call "DragDropCustomize.vi"("Function"=enum16{"Event", "Cleanup"}."Event", "CtlRef"=w704, "Event Type"=w705) -> ()  [unwired: 4 in, 5 out]
      }
      event "Tree": Item Close; "Tree": event #0x1e {
        n226 = event-data() -> ("Type"=w717:T12, "CtlRef"=w716:refnum<vi>, "Tag"=w715:string)  [unwired: 1 in, 2 out]
        n227 = case shown="\"Tree Item Open\"" w717 {
          tunnel: [14 15] -> w710
          tunnel: [15 14] -> w714
          frame "Tree Item Close", Default {
          }
          frame "Tree Item Open" {
          }
        }
        n228 = property class="Tree (strict)"(reference=w716, "Active Item Tag"=w715) -> (reference out=w711:refnum<vi>, "Glyph"=w713:i32)  [unwired: 1 in, 1 out]
        n229 = Equal?(x=w714, y=w713) -> (x = y?=w712:bool)
        n230 = case shown="True" w712 {
          tunnel: w711 -> [_ w720]
          tunnel: w710 -> [_ w719]
          tunnel: [_ w718] -> w707
          frame False {
          }
          frame True {
            n231 = property class="Tree (strict)"(reference=w720, "Glyph"=w719) -> (error out=w718:errorcluster)  [unwired: 1 in, 1 out]
          }
        }
        n232 = Enqueue Element(queue=w709, element="Save NEVER", error in (no error)=w707) -> ()  [unwired: 1 in, 3 out]
      }
      event "Tree": Edit Cell? {
        n233 = event-data() -> ("Col"=w726:i32)  [unwired: 1 in]
        n234 = Not Equal To 0?(x=w726) -> (x != 0?=w725:bool)
        n235 = event-data("Discard?"=w725) -> ()  [unwired: 2 in, 1 out]
      }
      event "Tree": Value Change; "Tree": Edit Cell {
        # "時刻を更新する"
        # "エディタ部へデータを送る"
        n236 = event-data() -> ("Type"=w733:T12)  [unwired: 1 in]
        n237 = case shown="\"Cell Edit\"" w733 {
          tunnel: w732 -> [w736 w739]
          tunnel: [w736 w745] -> w731
          tunnel: w729 -> [w734 w742]
          tunnel: w728 -> [_ w740]
          tunnel: w727 -> [_ w738]
          frame Default {
            n238 = Enqueue Element(queue=w734, element="Save NEVER") -> ()  [unwired: 2 in, 3 out]
          }
          frame "Cell Edit" {
            # "Store Undo Entry"
            n239 = call "StoreUndoEntry.vi"("editor refs"=w738, "Tree"=w739, "UndoBuffer"=w740) -> ("error out"=w737:errorcluster)  [unwired: 8 in]
            n240 = local read "Tree"() -> (w748:string)
            n241 = Format Date/Time String(time format string (%c)="%Y-%m-%d %H:%M:%S") -> (date/time string=w746:string)  [unwired: 2 in]
            n242 = property class="Tree (strict)"(reference=w739, error in=w737, "Active Item Tag"=w748, "ActiveColNum"=2 ("Active Cell:Active Column Number"), "Cell String"=w746) -> (reference out=w745:refnum<vi>, error out=w744:errorcluster)
            n243 = call <vilib>:"Clear Errors.vi"("error in (no error)"=w744) -> ("error out"=w741:errorcluster)  [unwired: 5 in, 1 out]
            n244 = Enqueue Element(queue=w742, element="Save EDIT", error in (no error)=w741) -> ()  [unwired: 1 in, 3 out]
          }
        }
        n245 = local read "editor refs"() -> (w730:refnum<vi>[])
        n246 = call "UpdateEditors.vi"("Array"=w730, "TreeControl in"=w731) -> ()  [unwired: 9 in, 1 out]
      }
      event "Title", "Description", "Script": Key Down? {
        # "キャレット位置を覚えておく"
        n247 = event-data() -> ("Char"=w755:i16, "VKey"=w752:T1, "CtlRef"=w757:refnum<vi>)  [unwired: 1 in]
        n248 = property class="Str"(reference=w757) -> ("Text.Selection"=→"Text.Selection":T2)  [unwired: 1 in, 2 out]
        n249 = Equal?(x=i16 8, y=w755) -> (x = y?=w753:bool)
        n250 = Select(t=eventvkey."Delete", s=w753, f=w752) -> (s? t:f=w750:T1)
        n251 = case shown="\"Enter\", \"Return\", \"Up\"..\"Right\", \"Home\"..\"PageDown\"" w750 {
          selector: w750 -> [_ _ _ _ w766]
          frame "Enter", "Return", "Up".."Right", "Home".."PageDown" {
            # "New undo context"
            n252 = local write "Last Modified"(refnum<vi> refnum ("Last Modified")) -> ()
          }
          frame "Shift".."Break", "Insert", "Escape".."Mute" {
            # "Do nothing"
          }
          frame "Delete" {
            n253 = local read "Edit Mode"() -> (w759:enum16{"unknown", "inserting", "deleting"})
            n254 = case shown="Default" w759 {
              frame Default {
                # "New undo context"
                n255 = local write "Last Modified"(refnum<vi> refnum ("Last Modified")) -> ()
                n256 = local write "Edit Mode"(enum16{"unknown", "inserting", "deleting"}."deleting" ("Edit Mode")) -> ()
              }
              frame "deleting" {
              }
            }
          }
          frame "ASCII", "Two Byte Char" {
            n257 = local read "Edit Mode"() -> (w762:enum16{"unknown", "inserting", "deleting"})
            n258 = case shown="Default" w762 {
              frame Default {
                # "New undo context"
                n259 = local write "Last Modified"(refnum<vi> refnum ("Last Modified")) -> ()
                n260 = local write "Edit Mode"(enum16{"unknown", "inserting", "deleting"}."inserting" ("Edit Mode")) -> ()
              }
              frame "inserting" {
              }
            }
          }
          frame Default {
            n261 = call "RaiseErrorIf.vi"("error message"="Unexpected key.") -> ()  [unwired: 10 in, 1 out]
            "VKey" <- w766
          }
        }
        n262 = event-data() -> ()  [unwired: 7 in, 1 out]
      }
      event "Title", "Description", "Script": Mouse Up {
        # "キャレット位置を覚えておく"
        n263 = event-data() -> ("CtlRef"=w768:refnum<vi>)  [unwired: 1 in]
        n264 = property class="Str"(reference=w768) -> ("Text.Selection"=w767:T2)  [unwired: 1 in, 2 out]
        n265 = local write "Text.Selection"(w767) -> ()
      }
      event "Title", "Description", "Script": Value Change {
        n266 = event-data() -> ("CtlRef"=w769:refnum<vi>)  [unwired: 1 in, 5 out]
        n267 = local write "Dirty"(w769) -> ()
      }
      event "Exec": Value Change {
        n268 = event-data() -> ("NewVal"=w771:bool)  [unwired: 1 in]
        n269 = case shown="True" w771 {
          tunnel: w770 -> [_ w775]
          frame False {
          }
          frame True {
            n270 = property on="Tree" class="Tree (strict)"() -> ("Value"=w772:string)  [unwired: 2 in, 2 out]
            n271 = Concatenate Strings("Execute " ("element"), w772) -> (w773:string)
            n272 = Enqueue Element(queue=w775, element=w773) -> ()  [unwired: 2 in, 3 out]
          }
        }
      }
      event "Tree": Double Click {
        n273 = event-data() -> ("Tag"=w776:string)  [unwired: 1 in]
        n274 = Concatenate Strings("Execute " ("element"), w776) -> (w777:string)
        n275 = case shown="Default" w776 {
          selector: w776 -> [_ w780]
          frame "" {
          }
          frame Default {
            # "ダブルクリックによる\nオープン・クローズは\n無効化する"
            n276 = invoke on="Tree" class="Tree (strict)" method="Navigate Tree.Get Child"("Tag"=w780) -> (error out=w781:errorcluster, "Navigate Tree:Get Child"=w782:string)  [unwired: 3 in, 2 out]
            n277 = case shown="No Error" w781 {
              tunnel: w782 -> [w784 _]
              tunnel: w780 -> [w783 _]
              frame No Error {
                n278 = case shown="Default" w784 {
                  tunnel: w783 -> [w790 _]
                  frame Default {
                    n279 = property on="Tree" class="Tree (strict)"("Active Item Tag"=w790) -> (error out=w787:errorcluster, "Open?"=w788:bool)  [unwired: 2 in, 1 out]
                    n280 = Not(x=w788) -> (.not. x?=w789:bool)
                    n281 = property on="Tree" class="Tree (strict)"(error in=w787, "Open?"=w789) -> (error out=w786:errorcluster)  [unwired: 1 in, 1 out]
                    n282 = control-ref of="Tree"() -> (w785:refnum<vi>)
                    n283 = call "OpenCloseSymbols.vi"("error in (no error)"=w786, "Tree ref"=w785) -> ()  [unwired: 8 in, 2 out]
                  }
                  frame "" {
                  }
                }
              }
              frame Error {
              }
            }
          }
        }
        n284 = Enqueue Element(queue=w778, element=w777) -> ()  [unwired: 2 in, 3 out]
      }
      event "VI Property Picker": Value Change {
        n285 = event-data() -> ("NewVal"=w791:bool)  [unwired: 1 in, 5 out]
        n286 = case shown="True" w791 {
          frame False {
          }
          frame True {
            n287 = Current VI's Path() -> (path=w804:path)
            n288 = Strip Path(path=w804) -> (stripped path=w803:path)  [unwired: 1 out]
            n289 = Build Path(base path=w803, name or relative path="VIPropertyPicker.vi") -> (appended path=w801:path)
            n290 = Open VI Reference(vi path=w801) -> (vi reference=w800:refnum<vi>, error out=w799:errorcluster)  [unwired: 5 in]
            n291 = invoke class="VI" method="FP.Open"(reference=w800, error in=w799, "Activate"=TRUE ("Activate?"), "State"=T4."Standard") -> (reference out=w796:refnum<vi>, error out=w794:errorcluster)  [unwired: 1 in, 3 out]
            n292 = property class="VI"(reference=w796, error in=w794) -> (reference out=w795:refnum<vi>, error out=w792:errorcluster, "Exec.State"=w793:T15)
            n293 = case shown="\"Idle\"" w793 {
              tunnel: w795 -> [_ w806]
              tunnel: w792 -> [_ w805]
              frame "Bad", Default {
              }
              frame "Idle" {
                n294 = invoke class="VI" method="Run VI"(reference=w806, error in=w805, "Wait until done"=FALSE ("Wait Until Done"), "Auto Dispose Ref"=TRUE ("Auto Dispose Reference")) -> ()  [unwired: 1 in, 5 out]
              }
            }
          }
        }
      }
    }
  }
  n295 = call "DragDropCustomize.vi"("Function"=enum16{"Event", "Cleanup"}."Cleanup", "error in (no error)"=w11) -> ()  [unwired: 5 in, 5 out]
